vi "BRig_dataTrial_sTrial_end.vi"() -> (2 "output_sTrial_end":i32)   [LabVIEW 2014]
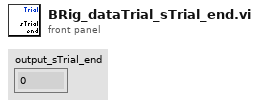
[diagram p1: front panel]
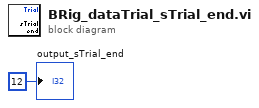
[diagram p0: block diagram]
diagram:
  "output_sTrial_end" <- 12 ("output_iBlock")
